vi "MES_Get Andon_Alarm Detail Messages.vi"(0 "StationName":string, 1 "LineNum":string, 5 "Main":string, 9 "VariableName":string, 11 "error in (no error)":errorcluster, 12 "Alarm":bool=TRUE, 13 "ColumonName  only Number string":string) -> (4 "Details Message":string, 6 "物料名称Array":string[](array[string]), 8 "Details Message Array":string[](array[string]), 15 "error out":errorcluster)   [LabVIEW 2017, in "SQLite.lvclass"]
doc: "查询每个工位的报警详细信息，此信息每个工位的具体报警，PLC需要提供报警表格。\nAndon报警，物料报警，质量报警，的信息都在此表格里面\n# daikinyi\n蒋松\njiangsong@outlook.com"
uses:
  SQLite.lvclass
  SQLiteFileName.ctl
  TabelFullName.ctl
  <vilib>/Utility/error.llb/Trim Whitespace.vi
  <userlib>/LabSQL/LabSQL.lvlib
  <userlib>/sushu/sushu.lvlib
panel:
  out "number (0 to 1)":dbl
  out "Select SQL CMD":string
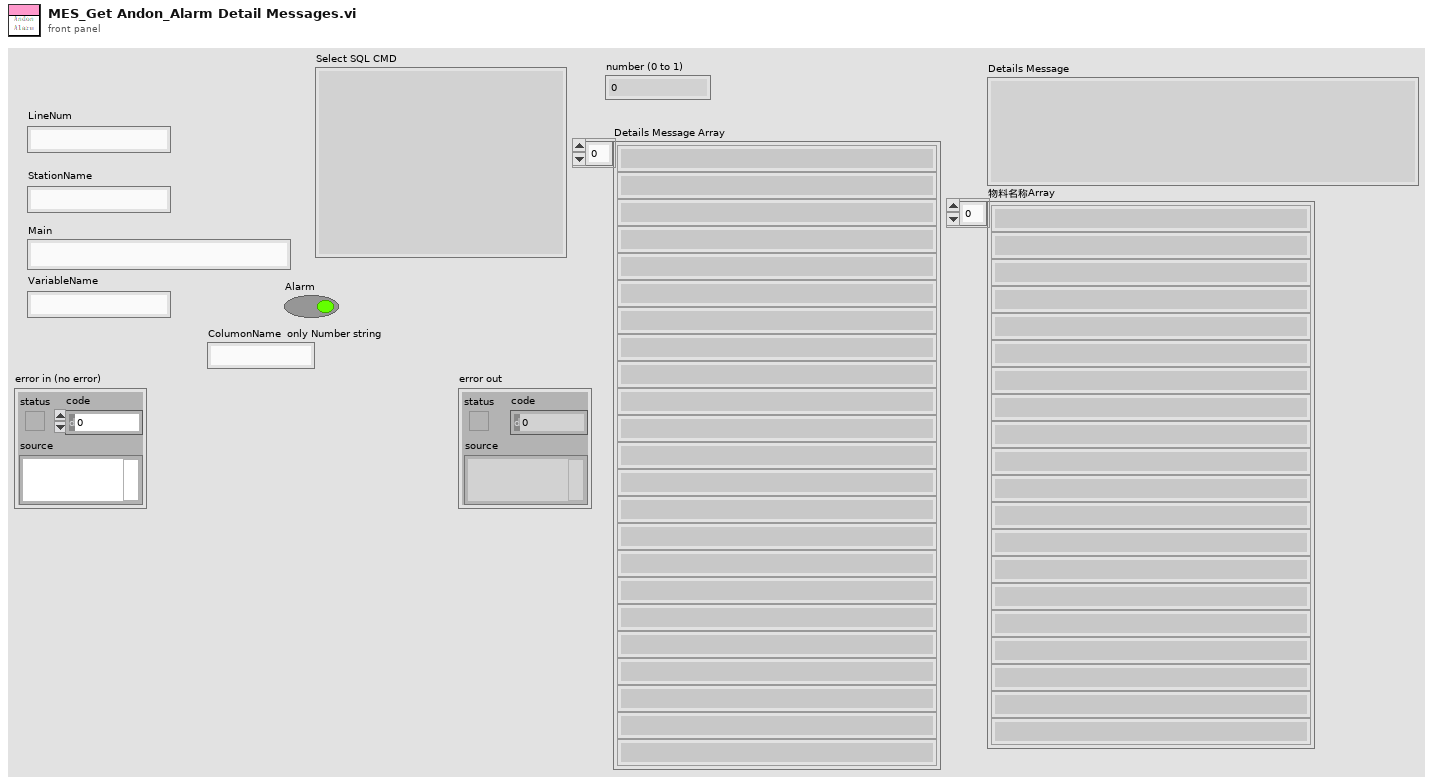
[diagram p1: front panel]
types:
  T1 = enum16{"Initialize", "Read", "Write", "UnInitialize"}
  T2 = typedef "SQLite.lvclass/TabelFullName.ctl" = string
  T3 = typedef "SQLite.lvclass/SQLiteFileName.ctl" = string
  T4 = cluster{"Current VI Reference":refnum<vi>, "Close Panel on Exit?":bool}
  T5 = cluster{"Core":cluster{"Current VI Reference":refnum<vi>, "Close Panel on Exit?":bool}, "VI Name":string}
  T6 = enum16{"Other", "SQL2008", "SQLite", "Access", "MySQL"}
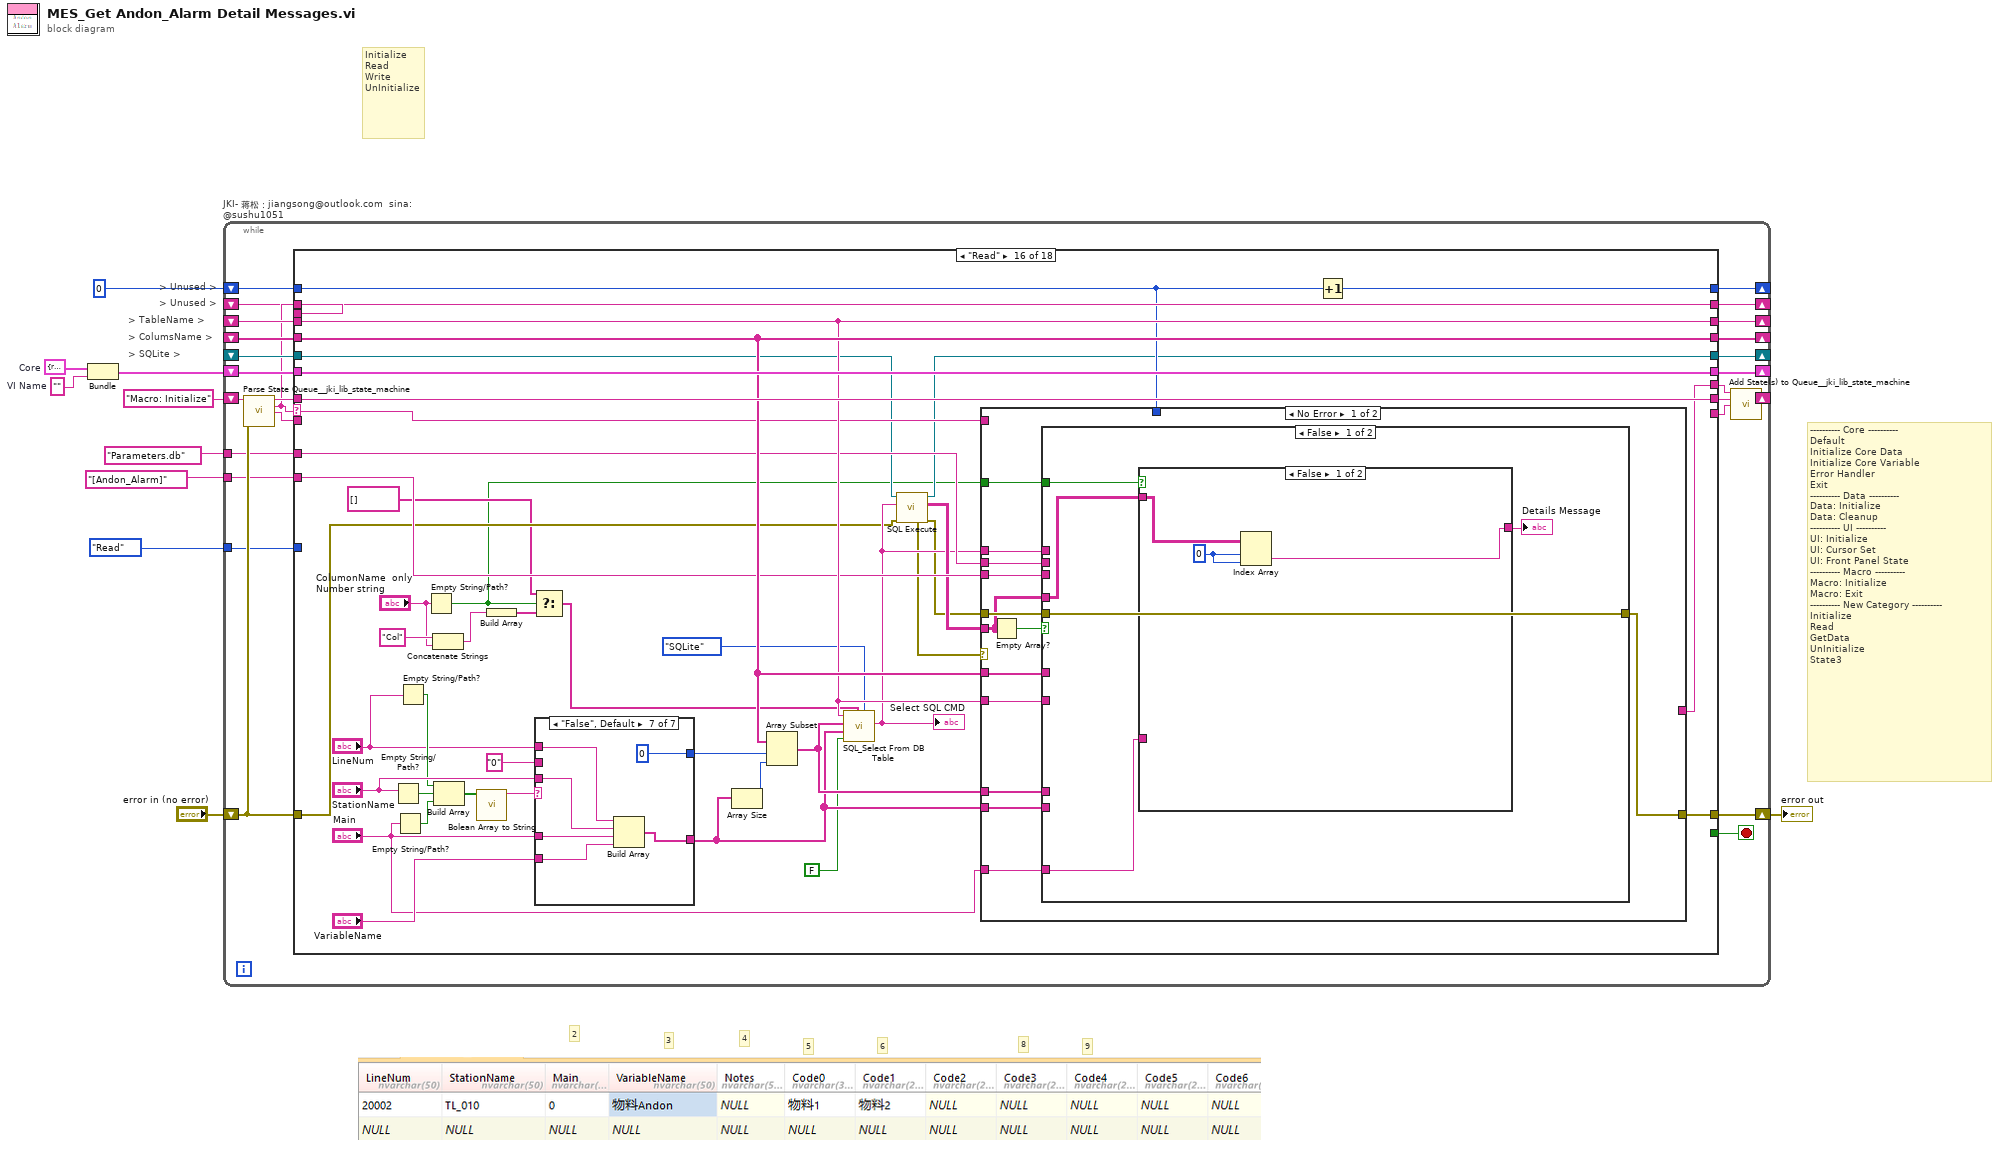
[diagram p0: block diagram]
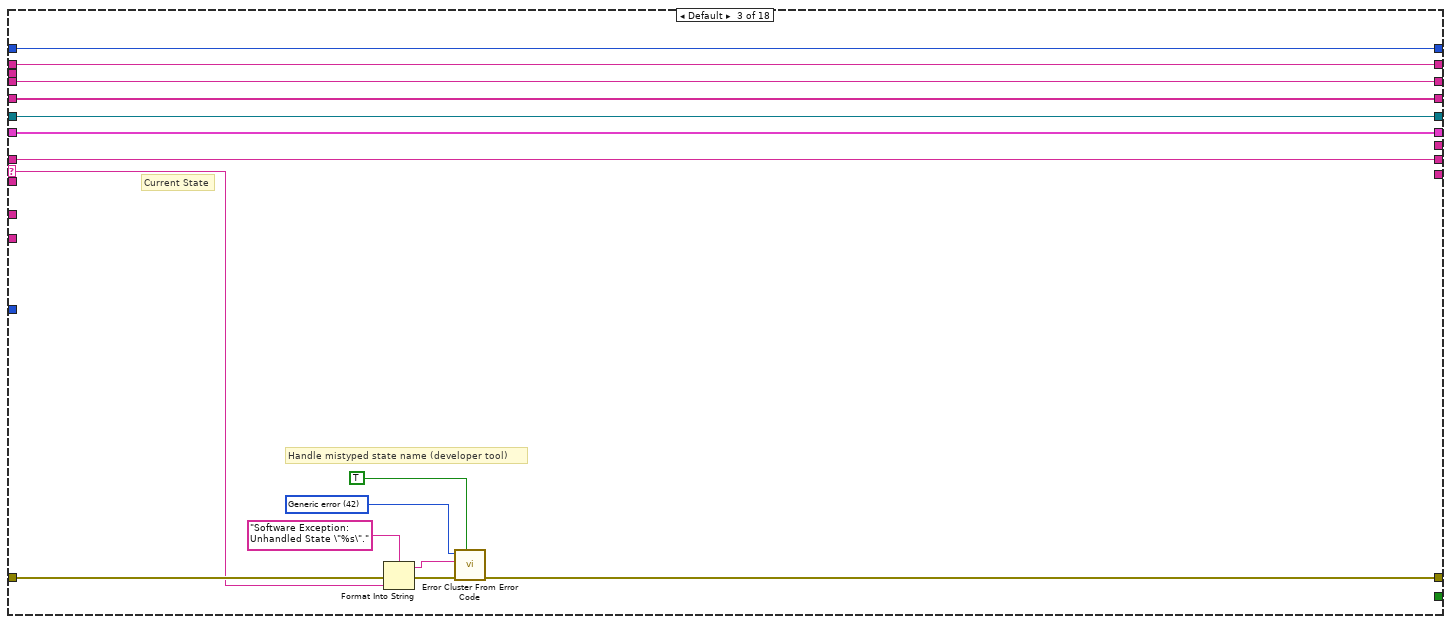
[diagram p4: hidden frame]
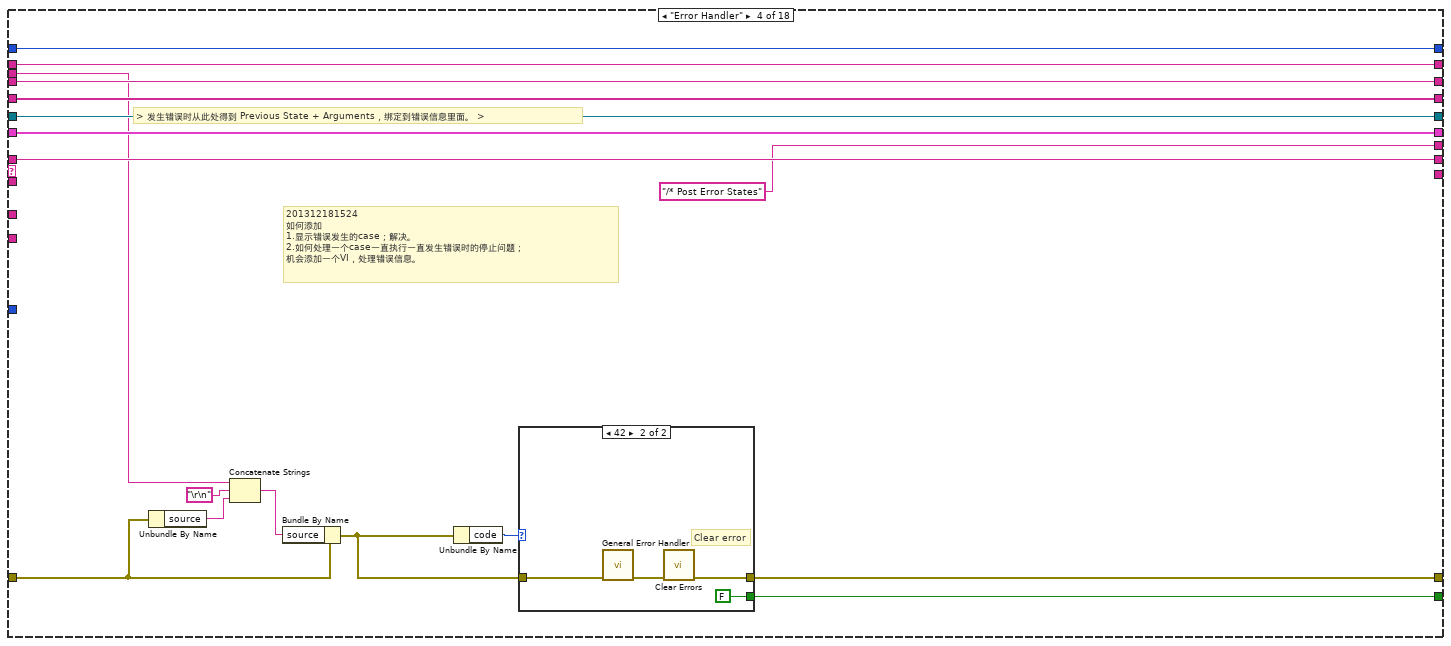
[diagram p5: hidden frame]
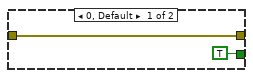
[diagram p6: hidden frame]
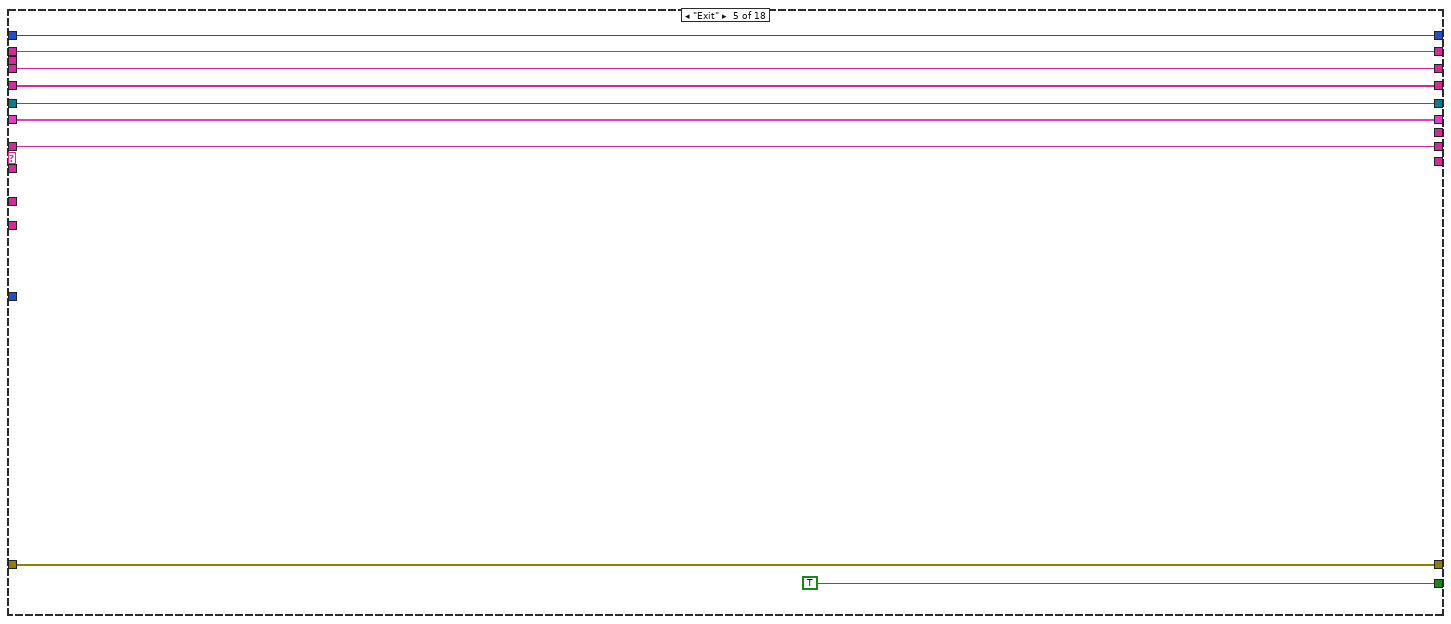
[diagram p7: hidden frame]
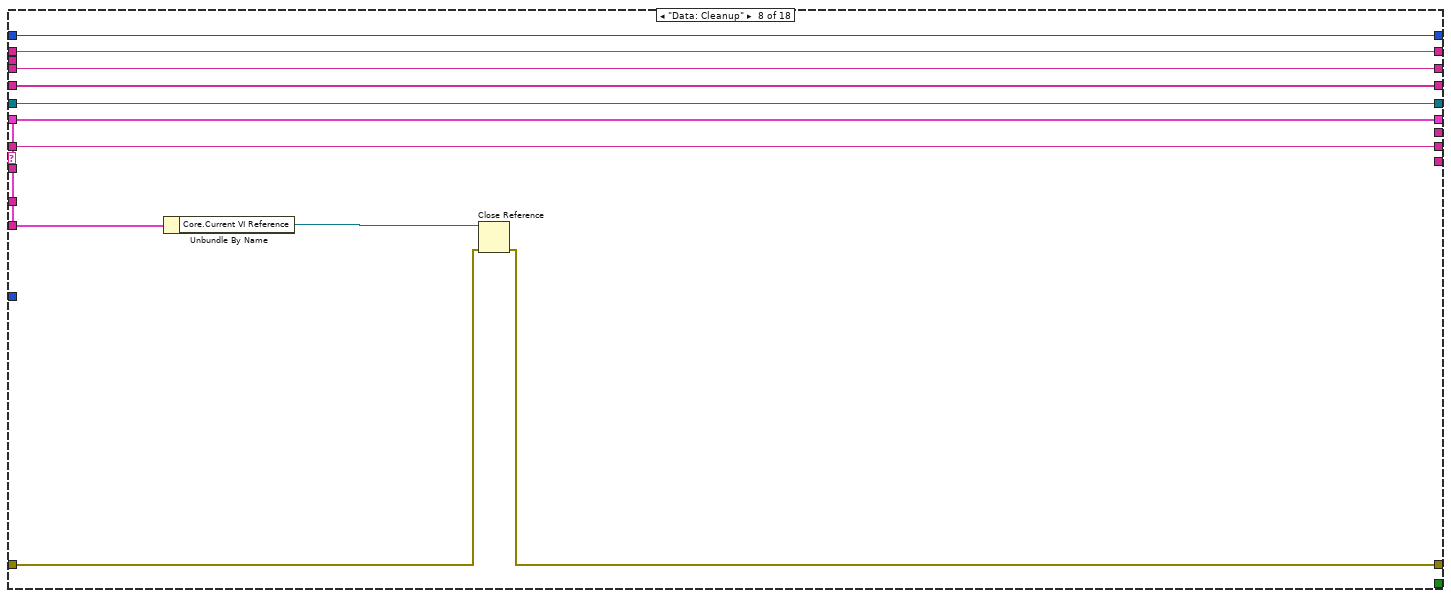
[diagram p10: hidden frame]
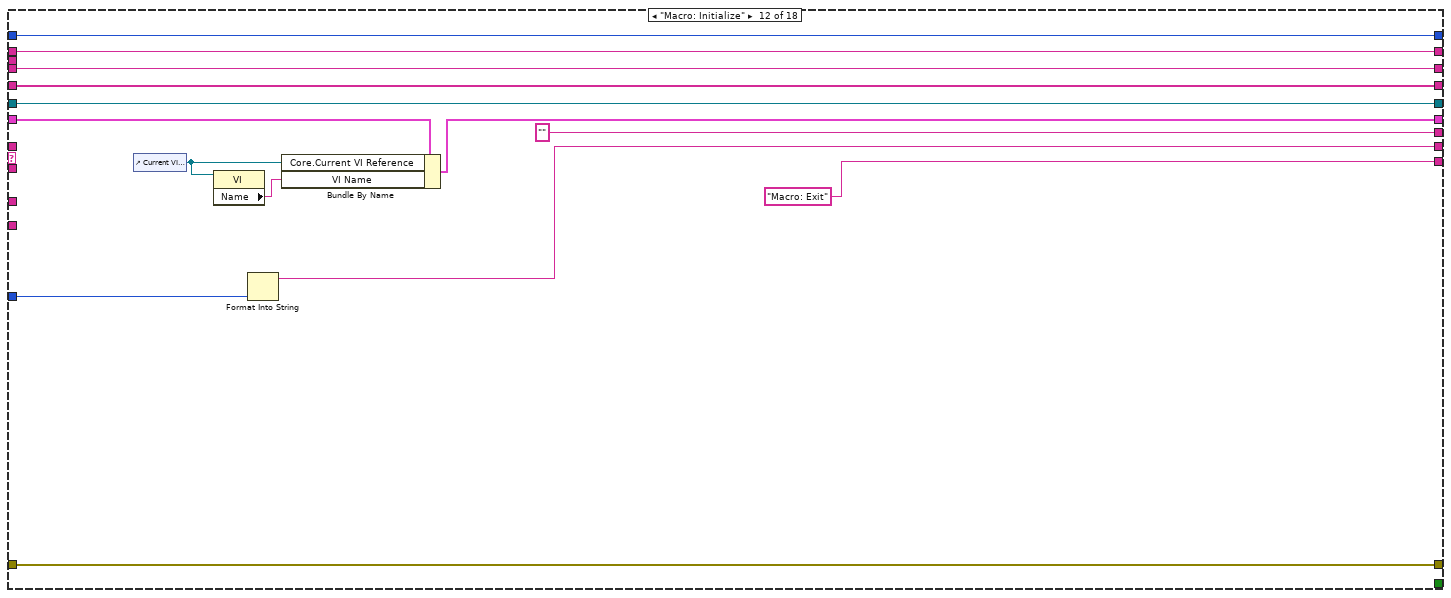
[diagram p14: hidden frame]
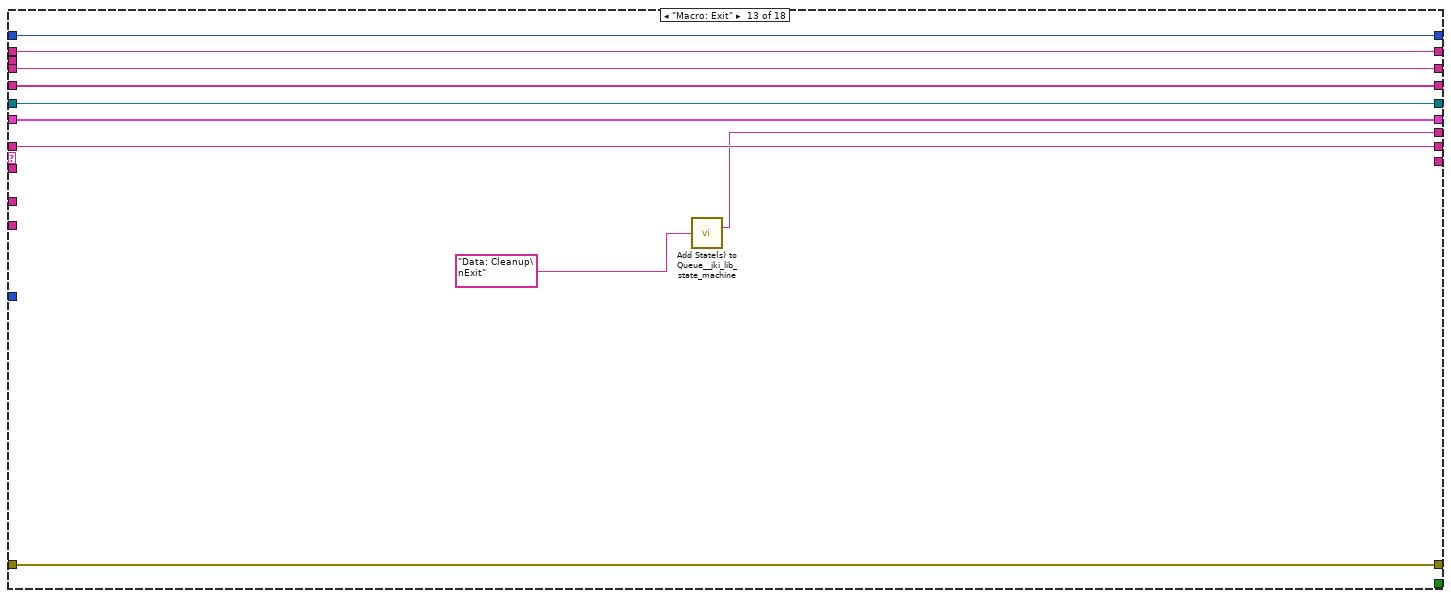
[diagram p15: hidden frame]
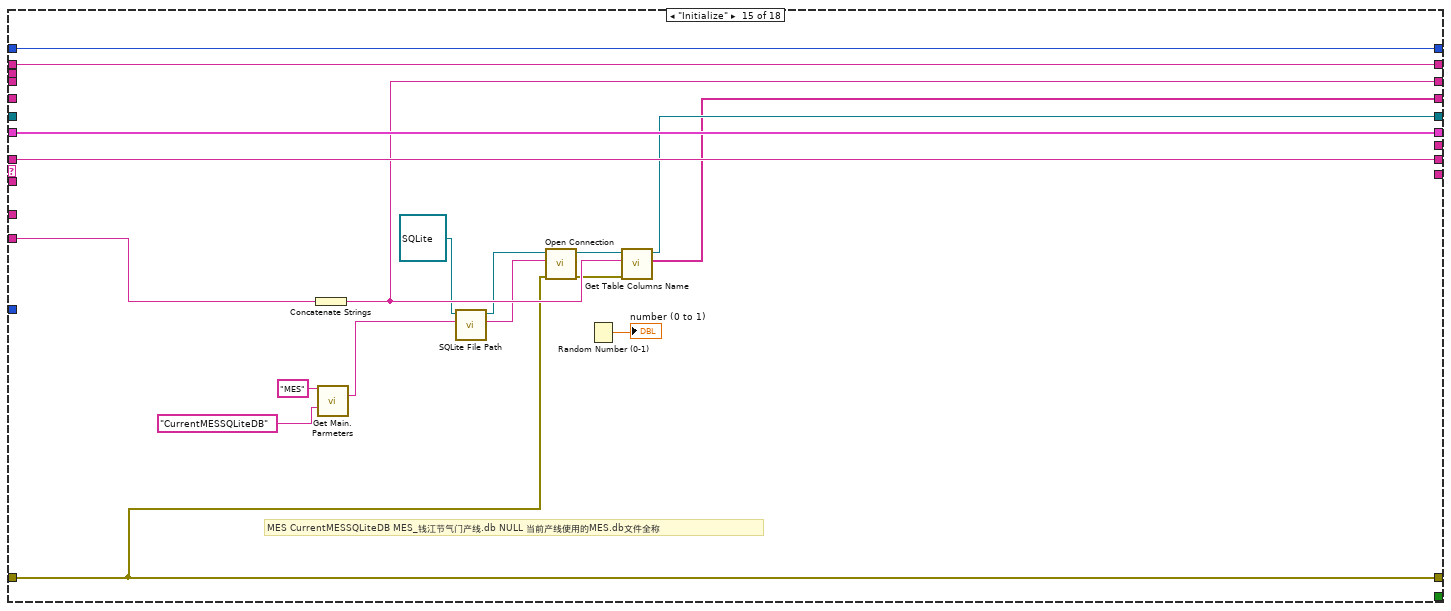
[diagram p17: hidden frame]
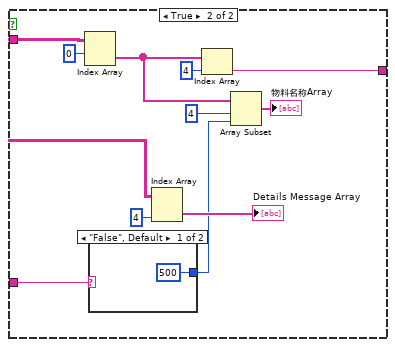
[diagram p18: hidden frame]
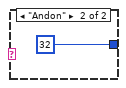
[diagram p19: hidden frame]
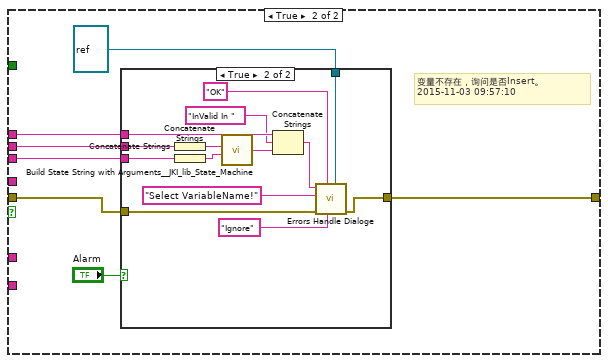
[diagram p20: hidden frame]
diagram:
  w10 = ""  # VI Name
  w9 = T4 {"Current VI Reference"=refnum, "Close Panel on Exit?"=FALSE}  # Core
  # "9"
  # "8"
  # "2"
  # "6"
  # "5"
  # "4"
  # "3"
  # "Initialize\nRead\nWrite\nUnInitialize"
  # "> Unused >"
  # "> SQLite >"
  # "> ColumsName >"
  # "> TableName >"
  # "> Unused >"
  # "---------- Core ----------\nDefault\nInitialize Core Data\nInitialize Core Variable\nError Handler\nExit\n---------- Data ----------\nData: Initialize\nData: Cleanup\n---------- UI ----------\nUI: Initialize\nUI: Cursor Set\nUI: Front Panel State\n---------- Macro ----------\nMacro: Initialize\nMacro: Exit\n---------- New Category ----------\nInitialize\nRead\nGetData\nUnInitialize\nState3"
  n1 = Bundle("Core"=w9, "VI Name"=w10) -> (w8:T5)  [unwired: 1 in]
  n2 = while "JKI- 蒋松：jiangsong@outlook.com  sina: @sushu1051" {
    shift-right: [w34] -> w3
    shift-left: "error in (no error)" -> [w32]
    shift-right: [w22] -> _
    shift-left: "Macro: Initialize" -> [w23]
    shift-right: [w29] -> _
    shift-left: _ -> [w31]
    shift-right: [w30] -> _
    shift-left: _ -> [w11]
    shift-right: [w24] -> _
    shift-left: w8 -> [w27]
    shift-right: [w25] -> _
    shift-left: _ -> [w18]
    shift-right: [w26] -> _
    shift-left: _ -> [w28]
    shift-right: [w17] -> _
    shift-left: 0 -> [w16]
    tunnel: T1."Read" ("CMD") -> [w15]
    tunnel: T3 "Parameters.db" ("SQLiteFileName") -> [w14]
    tunnel: T2 "[Andon_Alarm]" ("TabelFullName") -> [w13]
    stop <- w33 stop-if-true
    n3 = call <vilib>:"Parse State Queue__jki_lib_state_machine.vi"("State Queue"=w23, "Error In (no error)"=w32) -> ("Remaining States"=w36:string, "Current State"=w12:string, "Arguments"=w35:string)  [unwired: 10 in, 1 out]
    n4 = case shown="\"Read\"" w12 {
      selector: w12 -> [_ _ w55 _ _ _ _ _ _ _ _ _ _ _ _ w226 _ _]
      tunnel: w36 -> [w44 w46 w54 w76 w92 w101 w110 w117 w127 w135 w143 _ w166 w175 w199 w240 w352 w362]
      tunnel: w35 -> [_ _ _ _ _ _ _ _ _ _ _ _ _ _ _ _ _ _]
      tunnel: [w43 w52 w56 w70 w94 w103 w112 w119 w129 w137 w145 w160 w170 w178 w189 w227 w345 w353] -> w34
      tunnel: w32 -> [w43 w52 w57 w80 w94 w103 w112 w120 w129 w137 w145 w160 w170 w178 w189 w219 w345 w354]
      tunnel: [w44 w46 w54 w76 w92 w101 w110 w117 w127 w135 w143 w151 w166 w175 w199 w240 w352 w362] -> w21
      tunnel: [_ _ _ w69 TRUE _ _ _ _ _ _ _ _ _ _ _ _ _] -> w33
      tunnel: w12 -> [w42 w51 w67 w84 w99 w107 w115 w125 w133 w141 w149 w163 w173 w181 w198 w228 w346 w361]
      tunnel: w31 -> [w41 w50 w66 w83 w98 w106 w114 w124 w132 w140 w148 w162 w172 w180 _ w231 w351 w360]
      tunnel: [w42 w51 w67 w84 w99 w107 w115 w125 w133 w141 w149 w163 w173 w181 w198 w228 w346 w361] -> w30
      tunnel: [w41 w50 w66 w83 w98 w106 w114 w124 w132 w140 w148 w162 w172 w180 w191 w231 w351 w360] -> w29
      tunnel: w28 -> [w40 w49 w65 w82 w97 w105 w113 w123 w131 w139 w147 w161 w171 w179 _ w232 w350 w359]
      tunnel: w18 -> [w38 w47 w64 w74 w93 w102 w111 w118 w128 w136 w144 w159 w167 w176 _ w223 w349 w356]
      tunnel: w27 -> [w39 w48 w63 w81 w96 w104 w108 w121 w130 w138 w146 w153 w168 w177 w197 w239 w348 w358]
      tunnel: [w40 w49 w65 w82 w97 w105 w113 w123 w131 w139 w147 w161 w171 w179 w192 w232 w350 w359] -> w26
      tunnel: [w38 w47 w64 w74 w93 w102 w111 w118 w128 w136 w144 w159 w167 w176 w193 w221 w349 w355] -> w25
      tunnel: [w39 w48 w63 w81 w96 w104 w108 w121 w130 w138 w146 w152 w168 w177 w197 w239 w348 w358] -> w24
      tunnel: [_ _ _ "/* Post Error States" _ _ _ _ _ _ _ "" w165 _ _ w225 _ _] -> w20
      tunnel: [_ _ _ _ _ _ _ _ _ _ _ "Macro: Exit" _ _ _ _ _ _] -> w19
      tunnel: w16 -> [w37 w45 w53 w73 w91 w100 w109 w116 w126 w134 w142 w158 w164 w174 w196 w224 w347 w357]
      tunnel: [w37 w45 w53 w73 w91 w100 w109 w116 w126 w134 w142 w158 w164 w174 w196 w238 w347 w357] -> w17
      tunnel: w15 -> [_ _ _ _ _ _ _ _ _ _ _ w150 _ _ _ _ _ _]
      tunnel: w14 -> [_ _ _ _ _ _ _ _ _ _ _ _ _ _ _ w229 _ _]
      tunnel: w13 -> [_ _ _ _ _ _ _ _ _ _ _ _ _ _ w194 w230 _ _]
      tunnel: w11 -> [_ _ _ w68 _ _ _ _ _ _ _ _ _ _ _ _ _ _]
      frame "Idle" {
      }
      frame "---------- Core ----------" {
      }
      frame Default {
        w59 = 42 items=["No error", "Argument error", "Memory is full", "Out of zone", "End of file", "File already open", "Generic file I/O error", "File not found", "File permission error", "Disk is full", "Duplicate path", "Too many files open", "System feature not enabled", "Resource file not found", "Cannot add resource", "Resource not found", "Image not found", "Image memory error", "Pen does not exist", "Config type invalid", "Config token not found", "Config parse error", "Config memory error", "Bad external code format", "Bad external code offset", "External code not present", "Null window", "Destroy window error", "Null menu", "Print aborted", "Bad print record", "Print driver error", "Windows error during printing", "Memory error during printing", "Print dialog error", "Generic print error", "Invalid device refnum", "Device not found", "Device parameter error", "Device unit error", "Cannot open device", "Device call aborted", "Generic error", "Cancelled by user", "Object ID too low", "Object ID too high", "Object not in heap", "Unknown heap", "Unknown object (invalid DefProc)", "Unknown object (DefProc not in table)", "Message out of range", "Invalid (null) method", "Unknown message", "Manager call not supported", "Bad address", "Network operation in progress", "Network operation timed out", "Connection is busy", "Network attribute not supported", "Network error", "Address in use", "System out of memory", "Connection aborted", "Connection refused", "Not connected", "Already connected", "Connection closed", "Initialization error (interapplication manager)", "Bad occurrence", "Wait on unbound occurrence handler", "Occurrence queue overflow", "Datalog type conflict", "Unused", "Unrecognized type (interapplication manager)", "Memory corrupt", "Failed to make temporary DLL", "Old CIN version", "Drag socket not found", "Failed to load drop-object", "Failed to register OLE object", "Failed to release OLE object", "Format specifier type mismatch", "Unknown format specifier", "Too few format specifiers", "Too many format specifiers", "Scan failed", "Newer CIN version", "Error converting to variant", "Runtime menu error", "Password tampered", "Variant attribute not found", "Incompatible variant data type", "Event data is not available", "Event Store is not present", "Occurrence is not found", "Event Queue is not created", "Event info is not available", "Refnum passed is NULL", "Error retrieving Class GUID", "Error retrieving CoClass GUID", "Error retrieving TypeLib GUID.", "Bad built application magic bytes.", "Specific driver is different from the specific driver associated with the Logical Name.", "There is no session opened to the class driver.", "Max Error", "MAX - Error with config objects", "MAX - Error loading configuration", "MAX - Group not supported"]
        # "Current State"
        # "Handle mistyped state name (developer tool)"
        n5 = Format Into String(format string="Software Exception: Unhandled State \"%s\"." ("message"), error in=w57, w55) -> (resulting string=w60:string, error out=w61:errorcluster)  [unwired: 1 in]
        n6 = call <vilib>:"Error Cluster From Error Code.vi"("show call chain? (False)"=TRUE, "error in (no error)"=w61, "error message (\"\")"=w60, "error code (0)"=w59) -> ("error out"=w56:errorcluster)  [unwired: 5 in]
      }
      frame "Error Handler" {
        # "> 发生错误时从此处得到 Previous State + Arguments，绑定到错误信息里面。 >"
        # "201312181524\n如何添加\n1.显示错误发生的case；解决。\n2.如何处理一个case一直执行一直发生错误时的停止问题；\n机会添加一个VI，处理错误信息。"
        # "Clear error"
        n7 = Unbundle By Name(w80) -> ("source"=w78:string)
        n8 = Concatenate Strings(w68, "\r\n", w78) -> (w77:string)
        n9 = Bundle By Name(cluster=w80, "source"=w77) -> (w71:errorcluster)
        n10 = Unbundle By Name(w71) -> ("code"=w72:i32)
        n11 = case shown="42" w72 {
          tunnel: [TRUE FALSE] -> w69
          tunnel: w71 -> [w86 w89]
          tunnel: [w86 w87] -> w70
          frame 0, Default {
          }
          frame 42 {
            n12 = call <vilib>:"General Error Handler.vi"("error in (no error)"=w89) -> ("error out"=w88:errorcluster)  [unwired: 10 in, 4 out]
            n13 = call <vilib>:"Clear Errors.vi"("error in (no error)"=w88) -> ("error out"=w87:errorcluster)  [unwired: 5 in, 1 out]
          }
        }
      }
      frame "Exit" {
      }
      frame "---------- Data ----------" {
      }
      frame "Data: Initialize" {
      }
      frame "Data: Cleanup" {
        n14 = Unbundle By Name(w121) -> ("Core.Current VI Reference"=w122:refnum<vi>)
        n15 = Close Reference(reference=w122, error in (no error)=w120) -> (error out=w119:errorcluster)
      }
      frame "---------- UI ----------" {
      }
      frame "UI: Initialize" {
      }
      frame "---------- Macro ----------" {
      }
      frame "Macro: Initialize" {
        n16 = control-ref of="Current VI Reference"() -> (w154:refnum<vi>)
        n17 = property class="VI"(reference=w154) -> ("Name"=w155:string)  [unwired: 1 in, 2 out]
        n18 = Format Into String(w150) -> (resulting string=w151:string)  [unwired: 3 in, 1 out]
        n19 = Bundle By Name(cluster=w153, "Core.Current VI Reference"=w154, "VI Name"=w155) -> (w152:T5)
      }
      frame "Macro: Exit" {
        n20 = call <vilib>:"Add State(s) to Queue__jki_lib_state_machine.vi"("State(s) at Back (\"\")"="Data: Cleanup\nExit") -> ("States Out"=w165:string)  [unwired: 14 in]
      }
      frame "---------- New Category ----------" {
      }
      frame "Initialize" {
        # "MES\tCurrentMESSQLiteDB\tMES_钱江节气门产线.db\tNULL\t当前产线使用的MES.db文件全称"
        n21 = Concatenate Strings(w194) -> (w191:string)
        n22 = call "Get Main.Parmeters.vi"("Main"="MES", "VariableName"="CurrentMESSQLiteDB" ("Main")) -> ("Value"=w182:string)  [unwired: 7 in, 6 out]
        n23 = call "SQLite File Path.vi"("SQLiteFileName"=w182, "SQLite in"=refnum<class "SQLite.lvclass"> refnum ("SQLite.lvclass")) -> ("string"=w188:string, "SQLite out"=w186:refnum<class "SQLite.lvclass">)  [unwired: 7 in, 1 out]
        n24 = call-dynamic "Open Connection.vi"("error in (no error)"=w189, "ConnectionString"=w188, "HostDB in"=w186) -> ("error out"=w190:errorcluster, "HostDB out"=w195:refnum<class "SQLite.lvclass">)  [unwired: 7 in]
        n25 = Random Number (0-1)() -> (number: 0 to 1=→"number (0 to 1)":dbl)
        n26 = call-dynamic "Get Table Columns Name.vi"("error in (no error)"=w190, "TableName"=w191, "HostDB in"=w195) -> ("ColunmsList"=w192:string[], "HostDB out"=w193:refnum<class "SQLite.lvclass">)  [unwired: 4 in, 3 out]
      }
      frame "Read" {
        n27 = Empty String/Path?(string/path="StationName") -> (empty?=w216:bool)
        n28 = Empty String/Path?(string/path="Main") -> (empty?=w215:bool)
        n29 = Empty String/Path?(string/path="LineNum") -> (empty?=w210:bool)
        n30 = Empty String/Path?(string/path="ColumonName  only Number string") -> (empty?=w200:bool)
        n31 = Concatenate Strings("Col" ("string"), "ColumonName  only Number string") -> (w203:string)
        n32 = Build Array(w210, w216, w215) -> (w214:bool[])
        n33 = call <userlib>:"Bolean Array to String.vi"("Bolean Array"=w214) -> ("Bolean String"=w213:string)  [unwired: 10 in]
        n34 = Build Array(w203) -> (w202:string[])
        n35 = Select(t=string[] [] ("SelectedColumnsNameList"), s=w200, f=w202) -> (s? t:f=w205:string[])
        n36 = case shown="\"False\", Default" w213 {
          tunnel: [w313 w317 w320 w326 w332 w338 w344] -> w235
          tunnel: "Main" -> [w312 w314 _ w323 _ w333 w343]
          tunnel: "VariableName" -> [w311 w316 w319 w325 w331 w337 w342]
          tunnel: "StationName" -> [w309 _ _ _ w328 w334 w341]
          tunnel: [1 ("index") 2 ("index") 3 ("index") 0 ("index") 0 ("index") 0 ("index") 0 ("index")] -> w211
          tunnel: "LineNum" -> [_ _ _ w321 w329 w335 w339]
          tunnel: "0" ("element") -> [_ _ _ w322 w327 _ _]
          frame "100" {
            n37 = Build Array(w309, w312, w311) -> (w313:string[])
          }
          frame "110" {
            n38 = Build Array(w314, w316) -> (w317:string[])
          }
          frame "111" {
            n39 = Build Array(w319) -> (w320:string[])
          }
          frame "010" {
            n40 = Build Array(w321, w322, w323, w325) -> (w326:string[])
          }
          frame "001" {
            n41 = Build Array(w329, w328, w327, w331) -> (w332:string[])
          }
          frame "000" {
            n42 = Build Array(w335, w334, w333, w337) -> (w338:string[])
          }
          frame "False", Default {
            n43 = Build Array(w339, w341, w343, w342) -> (w344:string[])
          }
        }
        n44 = Array Size(array=w235) -> (size(s)=w234:i32)
        n45 = Array Subset(array=w232, index=w211, length=w234) -> (w237:string[])
        n46 = call <userlib>:"SQL_Select From DB Table.vi"("DB Type"=T6."SQLite", "SelectedColumnsNameList"=w205, "Check ASCII?"=FALSE, "ColumnsValue"=w235, "ColumnsNameList"=w237, "TableName"=w231) -> ("Select SQL CMD"=w220:string)  [unwired: 5 in]
        "Select SQL CMD" <- w220
        n47 = call-dynamic "SQL Execute.vi"("error in (no error)"=w219, "Command Text"=w220, "HostDB in"=w223) -> ("error out"=w218:errorcluster, "Table Control"=w222:string[][], "HostDB out"=w221:refnum<class "SQLite.lvclass">)  [unwired: 4 in, 2 out]
        n48 = case shown="No Error" w218 {
          selector: w218 -> [_ w301]
          tunnel: w237 -> [w253 _]
          tunnel: w218 -> [w252 w308]
          tunnel: w220 -> [w250 _]
          tunnel: w222 -> [w249 _]
          tunnel: w235 -> [w248 _]
          tunnel: w232 -> [w247 _]
          tunnel: w231 -> [w246 _]
          tunnel: w230 -> [w245 _]
          tunnel: w229 -> [w244 _]
          tunnel: [w243 w307] -> w227
          tunnel: w226 -> [_ w300]
          tunnel: [_ w299] -> w225
          tunnel: w224 -> [_ w298]
          tunnel: "Main" -> [w242 _]
          tunnel: w200 -> [w241 _]
          frame No Error {
            n49 = Empty Array?(array=w249) -> (empty?=w251:bool)
            n50 = case shown="False" w251 {
              tunnel: [w258 w280] -> w243
              tunnel: w247 -> [_ _]
              tunnel: w246 -> [_ _]
              tunnel: w248 -> [_ _]
              tunnel: w253 -> [_ _]
              tunnel: w252 -> [w258 w281]
              tunnel: w250 -> [_ w277]
              tunnel: w244 -> [_ w279]
              tunnel: w245 -> [_ w278]
              tunnel: w249 -> [w256 _]
              tunnel: w242 -> [w255 _]
              tunnel: w241 -> [w254 _]
              frame False {
                n51 = case shown="False" w254 {
                  tunnel: [w259 w270] -> w257
                  tunnel: w256 -> [w261 w266]
                  tunnel: w255 -> [_ w263]
                  frame False {
                    w260 = 0 ("index (row)")
                    n52 = Index Array(array=w261, index (row)=w260, index (col)=w260) -> (element=w259:string)
                  }
                  frame True {
                    n53 = Index Array(array=w266, index (row)=0) -> (element=w269:string[])  [unwired: 1 in]
                    n54 = case shown="\"False\", Default" w263 {
                      tunnel: [500 ("length") 32 ("length")] -> w262
                      frame "False", Default {
                      }
                      frame "Andon" {
                      }
                    }
                    n55 = Index Array(array=w266, index (col)=4 ("disabled index (col)")) -> (element=→"Details Message Array":string[])  [unwired: 1 in]
                    n56 = Index Array(array=w269, index=4) -> (element=w270:string)
                    n57 = Array Subset(array=w269, index=4, length=w262) -> (→"物料名称Array":string[])
                  }
                }
                "Details Message" <- w257
              }
              frame True {
                # "变量不存在，询问是否Insert。\n2015-11-03 09:57:10"
                n58 = case shown="True" "Alarm" {
                  tunnel: w281 -> [w282 w296]
                  tunnel: [w282 w295] -> w280
                  tunnel: w279 -> [_ w294]
                  tunnel: w278 -> [_ w293]
                  tunnel: w277 -> [_ w292]
                  tunnel: refnum<vi> refnum ("VI Ref") -> [_ w283]
                  frame False {
                  }
                  frame True {
                    n59 = Concatenate Strings(w294) -> (w291:string)
                    n60 = Concatenate Strings(w293) -> (w290:string)
                    n61 = call <vilib>:"Build State String with Arguments__JKI_lib_State_Machine.vi"("Arguments (\"\")"=w290, "State"=w291) -> ("State with Arguments"=w288:string)  [unwired: 4 in]
                    n62 = Concatenate Strings(w292, "InValid In " ("Message"), w288) -> (w287:string)
                    n63 = call <userlib>:"Errors Handle Dialoge.vi"("VI Ref"=w283, "Cancel Text"="Ignore", "OK Text"="OK", "error in (no error)"=w296, "Title Text"="Select VariableName!", "Message"=w287) -> ("error out"=w295:errorcluster)  [unwired: 4 in, 1 out]
                  }
                }
              }
            }
          }
          frame Error {
            n64 = call <vilib>:"Clear Errors.vi"("error in (no error)"=w308) -> ("error out"=w307:errorcluster)  [unwired: 5 in, 1 out]
            n65 = Unbundle By Name(w301) -> ("status"=w297:bool)
            n66 = Equal To 0?(x=w298) -> (x = 0?=w305:bool)
            n67 = And(x=w297, y=w305) -> (x .and. y?=w304:bool)
            n68 = call <vilib>:"Add State(s) to Queue__jki_lib_state_machine.vi"("State(s) in Front (\"\")"="Initialize" ("Remaining States"), "State(s) in (\"\")"=w300) -> ("States Out"=w302:string)  [unwired: 13 in]
            n69 = Select(t=w302, s=w304, f="GetData") -> (s? t:f=w299:string)
          }
        }
        n70 = Increment(x=w224) -> (x+1=w238:i32)
      }
      frame "GetData" {
      }
      frame "UnInitialize" {
        n71 = call-dynamic "Close Connection.vi"("error in (no error)"=w354, "HostDB in"=w356) -> ("error out"=w353:errorcluster, "HostDB out"=w355:refnum<class "SQLite.lvclass">)  [unwired: 8 in]
      }
    }
    n72 = call <vilib>:"Add State(s) to Queue__jki_lib_state_machine.vi"("State(s) in Front (\"\")"=w20, "State(s) in (\"\")"=w21, "State(s) at Back (\"\")"=w19) -> ("States Out"=w22:string)  [unwired: 12 in]
  }
  "error out" <- w3
